vi "Alarma_Timer_&_MsgEvento.vi"(11 "MOTIVO":string) -> ()   [LabVIEW 2018]
uses:
  Global/TimerReferences.vi
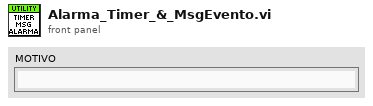
[diagram p1: front panel]
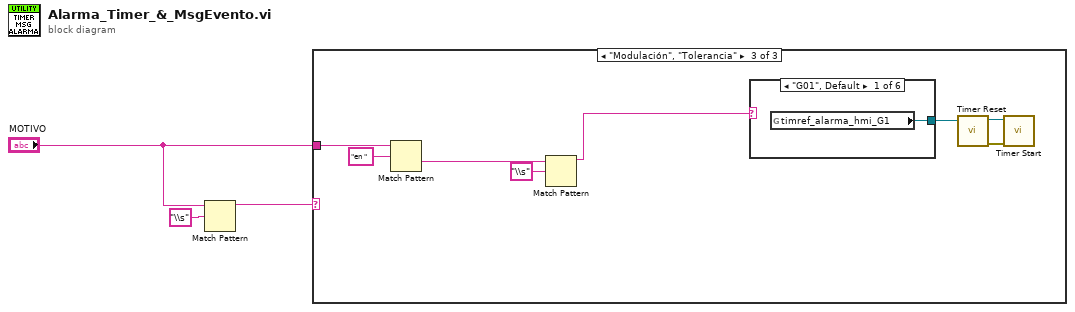
[diagram p0: block diagram]
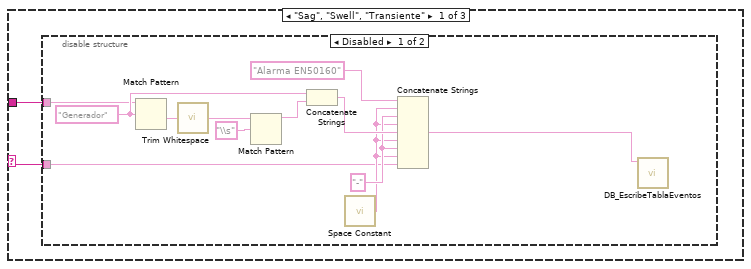
[diagram p2: hidden frame]
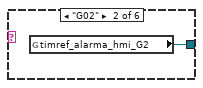
[diagram p5: hidden frame]
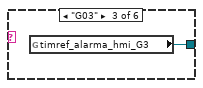
[diagram p6: hidden frame]
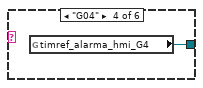
[diagram p7: hidden frame]
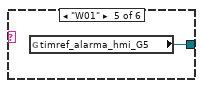
[diagram p8: hidden frame]
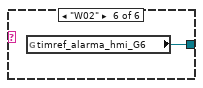
[diagram p9: hidden frame]
diagram:
  n1 = Match Pattern(string="MOTIVO", regular expression="\\s") -> (before substring=w1:string)  [unwired: 1 in, 3 out]
  n2 = case shown="\"Modulación\", \"Tolerancia\"" w1 {
    selector: w1 -> [w4 _ _]
    tunnel: "MOTIVO" -> [w5 _ w23]
    frame "Sag", "Swell", "Transiente" {
      n3 = disable-structure shown="Disabled" {
        disable-tunnel: w5 -> [w11 _]
        disable-tunnel: w4 -> [w7 _]
        frame Disabled {
          w9 = "-" ("regular expression")
          w14 = "Generador" ("regular expression")
          n4 = Match Pattern(string=w11, regular expression=w14) -> (after substring=w17:string)  [unwired: 1 in, 3 out]
          n5 = call <vilib>:"Trim Whitespace.vi"("string"=w17) -> ("trimmed string"=w16:string)  [unwired: 1 in]
          n6 = Match Pattern(string=w16, regular expression="\\s") -> (before substring=w13:string)  [unwired: 1 in, 3 out]
          n7 = Concatenate Strings(w14, w13) -> (w10:string)
          n8 = call <vilib>:"Space Constant.vi"() -> ("String"=w8:string)
          n9 = Concatenate Strings("Alarma EN50160" ("string"), w8, w9, w8, w10, w8, w9, w8, w7) -> (w6:string)
          n10 = call "DB_EscribeTablaEventos.vi"("DESCRIPCION"=w6) -> ()  [unwired: 10 in, 1 out]
        }
        frame Enabled {
        }
      }
    }
    frame Default {
    }
    frame "Modulación", "Tolerancia" {
      n11 = Match Pattern(string=w23, regular expression="en ") -> (after substring=w19:string)  [unwired: 1 in, 3 out]
      n12 = Match Pattern(string=w19, regular expression="\\s") -> (before substring=w18:string)  [unwired: 1 in, 3 out]
      n13 = case shown="\"G01\", Default" w18 {
        tunnel: [w26 w27 w28 w29 w30 w31] -> w22
        frame "G01", Default {
          n14 = global read "TimerReferences.vi" "timref_alarma_hmi_G1"() -> (w26:refnum<data-value>)
        }
        frame "G02" {
          n15 = global read "TimerReferences.vi" "timref_alarma_hmi_G2"() -> (w27:refnum<data-value>)
        }
        frame "G03" {
          n16 = global read "TimerReferences.vi" "timref_alarma_hmi_G3"() -> (w28:refnum<data-value>)
        }
        frame "G04" {
          n17 = global read "TimerReferences.vi" "timref_alarma_hmi_G4"() -> (w29:refnum<data-value>)
        }
        frame "W01" {
          n18 = global read "TimerReferences.vi" "timref_alarma_hmi_G5"() -> (w30:refnum<data-value>)
        }
        frame "W02" {
          n19 = global read "TimerReferences.vi" "timref_alarma_hmi_G6"() -> (w31:refnum<data-value>)
        }
      }
      n20 = call "Timer Reset.vi"("Timer reference"=w22) -> ("error out"=w21:errorcluster, "Timer reference  out"=w20:refnum<data-value>)  [unwired: 9 in]
      n21 = call "Timer Start.vi"("error in (no error)"=w21, "Timer reference"=w20) -> ()  [unwired: 8 in, 2 out]
    }
  }
